vi "Add Header.vi"(8 "error in (no error)":errorcluster, 9 "Value":string, 10 "Name":string, 11 "HTTPHeaders_NET in":refnum<class "HttpHeaders_NET.lvclass">) -> (0 "error out":errorcluster, 3 "HTTPHeaders_NET out":refnum<class "HttpHeaders_NET.lvclass">)   [LabVIEW 2018, in "HttpClient_NET.lvlib" / "HttpHeaders_NET.lvclass"]
uses:
  HttpHeaders_NET.lvclass
  HttpHeaders_NET.lvclass/HttpHeaders_NET.ctl
  System.Net.Http
  Accessors/Read NET_HttpHeaders.vi
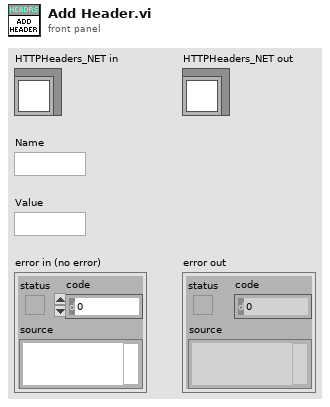
[diagram p1: front panel]
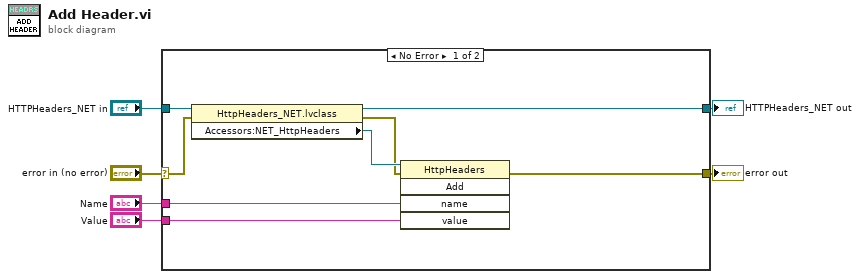
[diagram p0: block diagram]
diagram:
  n1 = case shown="No Error" "error in (no error)" {
    selector: "error in (no error)" -> [w9 w16]
    tunnel: [w7 w16] -> w5
    tunnel: [w13 w15] -> w3
    tunnel: "HTTPHeaders_NET in" -> [w14 w15]
    tunnel: "Name" -> [w11 _]
    tunnel: "Value" -> [w10 _]
    frame No Error {
      n2 = property class="HttpHeaders_NET.lvclass"(reference=w14, error in=w9) -> (reference out=w13:refnum<class "HttpHeaders_NET.lvclass">, error out=w8:errorcluster, "Accessors:NET_HttpHeaders"=w12:refnum<k24>)
      n3 = invoke class="HttpHeaders" method="Add"(reference=w12, error in=w8, "name"=w11, "value"=w10) -> (error out=w7:errorcluster)  [unwired: 1 in, 4 out]
    }
    frame Error {
    }
  }
  "error out" <- w5
  "HTTPHeaders_NET out" <- w3
